vi "MB Ethernet Slave Protocol Write.vi"(8 "error in (no error)":errorcluster, 9 "timeout":i32=10000, 10 "data":u8[](array[numeric]), 11 "protocol layer in":refnum<class "TCP Slave.lvclass">) -> (0 "error out":errorcluster, 1 "timed out?":bool, 3 "protocol layer out":refnum<class "TCP Slave.lvclass">)   [LabVIEW 2019, in "NI_modbus_upd.lvlib"]
doc: "Writes to the established TCP connection stored in the class."
uses:
  NI_modbus_upd.lvlib
  <vilib>/Modbus/subvis/Protocol/TCP/TCP Shared Components/TCP Shared Components.lvlib
  <vilib>/Modbus/subvis/Protocol/TCP/TCP Slave/TCP Slave.lvclass
  C:/Program Files (x86)/National Instruments/LabVIEW 2019/vi.lib/Modbus/subvis/Protocol/Interfaces/Network Slave/Network Slave.lvclass
  C:/Program Files (x86)/National Instruments/LabVIEW 2019/vi.lib/Modbus/subvis/Protocol/Interfaces/Network Protocol/Network Protocol.lvclass
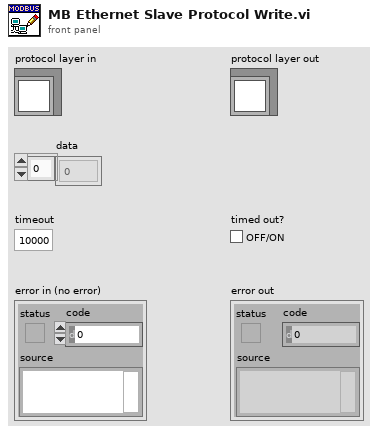
[diagram p1: front panel]
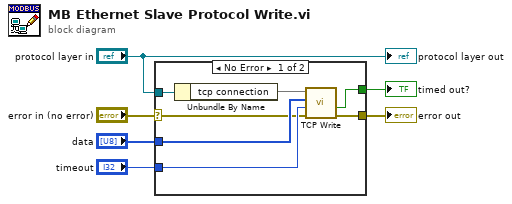
[diagram p0: block diagram]
diagram:
  n1 = case shown="No Error" "error in (no error)" {
    selector: "error in (no error)" -> [w7 w14]
    tunnel: "protocol layer in" -> [w13 _]
    tunnel: "data" -> [w11 _]
    tunnel: "timeout" -> [w10 _]
    tunnel: [w9 w14] -> w3
    tunnel: [w8 _] -> w2
    frame No Error {
      n2 = Unbundle By Name(w13) -> ("tcp connection"=w12)
      n3 = call <vilib>:"TCP Write.vi"("error in (no error)"=w7, "timeout"=w10, "data"=w11, "connection ID"=w12) -> ("error out"=w9:errorcluster, "timed out?"=w8:bool)  [unwired: 6 in]
    }
    frame Error {
    }
  }
  "error out" <- w3
  "timed out?" <- w2
  "protocol layer out" <- "protocol layer in"
